vi "Actividad Extra 13 (2).vi"() -> ()   [LabVIEW 2018]
uses:
  ControlExtraTrece.ctl
panel:
  out "Toluca":bool
  out "Zinacantepec":bool
  out "Capultitlan":bool
  out "Metepec":bool
  out "San Mateo":bool
  out "KM RECORRIDOS":i32
  out "DINERO RESTANTE":i32
  out "MUNICIPIO ACTUAL":T1
  in  "Detener Recorrido":bool
  in  "Y":i32
  in  "X":i32
  # "RECORRIDO POR MUNICIPIOS"
  # "COORDENADAS"
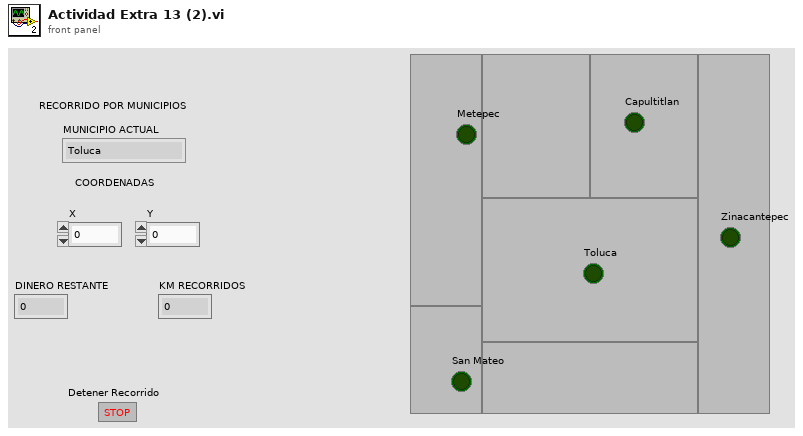
[diagram p1: front panel]
types:
  T1 = typedef "ControlExtraTrece.ctl" = enum16{"Toluca", "Metepec", "Zinacantepec", "San Mateo Atenco", "Capultitlan"}
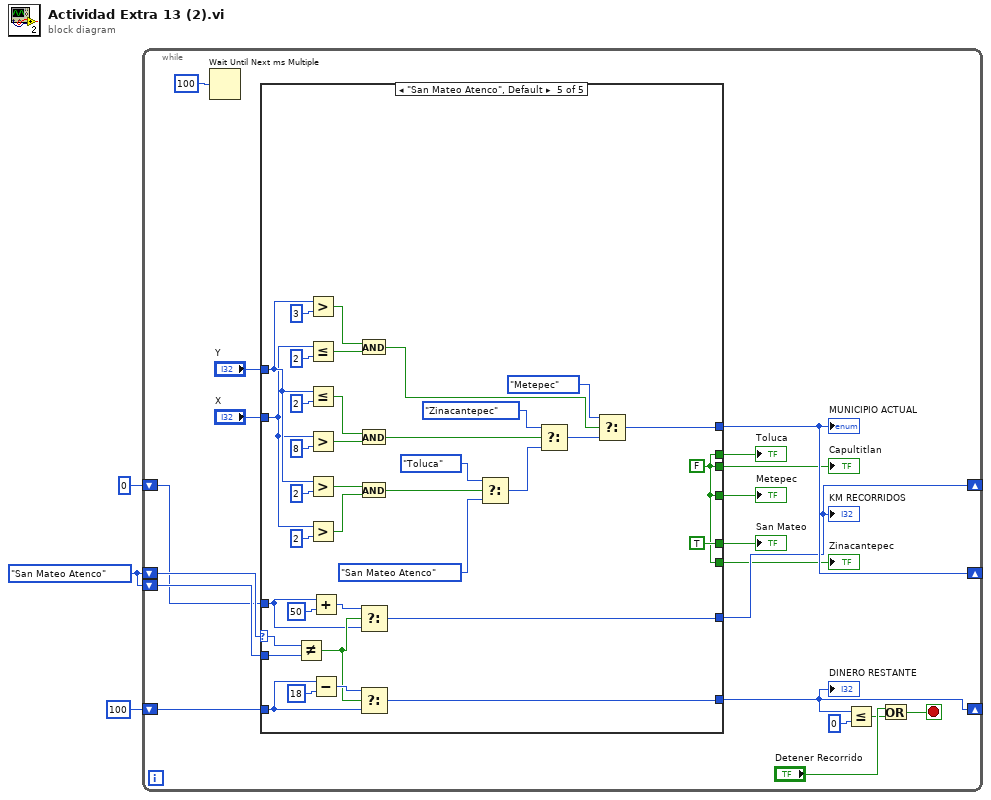
[diagram p0: block diagram]
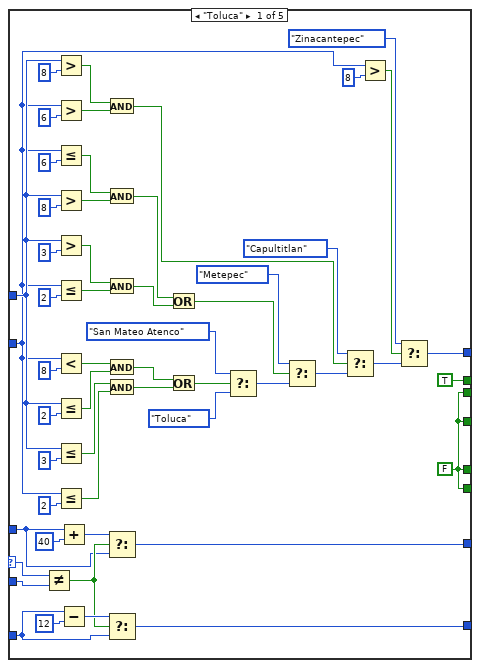
[diagram p2: hidden frame]
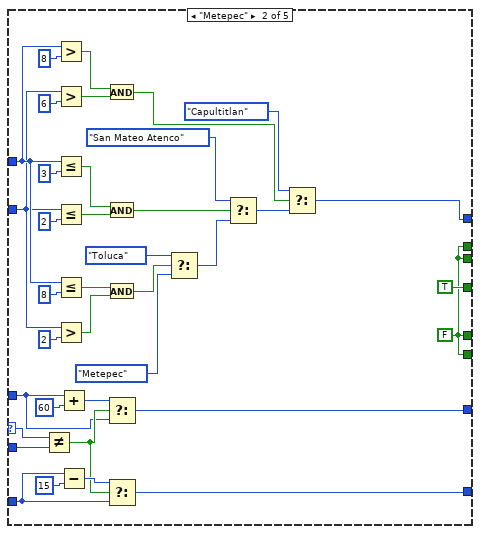
[diagram p3: hidden frame]
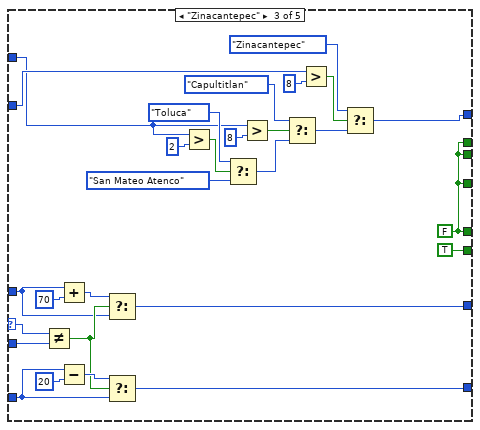
[diagram p4: hidden frame]
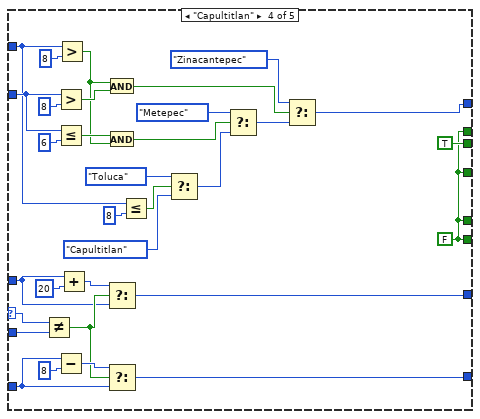
[diagram p5: hidden frame]
diagram:
  w3 = ControlExtraTrece."San Mateo Atenco"
  n1 = while {
    shift-right: [w20] -> _
    shift-left: w3 -> [w22]
    shift-left: w3 -> [w17]
    shift-right: [w10] -> _
    shift-left: 100 -> [w16]
    shift-right: [w14] -> _
    shift-left: 0 -> [w15]
    stop <- w12 stop-if-true
    n2 = Wait Until Next ms Multiple(millisecond multiple=u32 100) -> ()  [unwired: 1 out]
    n3 = case shown="\"San Mateo Atenco\", Default" w22 {
      selector: w22 -> [w25 w78 w116 w144 w175]
      tunnel: [w72 w107 w138 w167 w204] -> w20
      tunnel: "Y" -> [w45 w96 w129 w157 w193]
      tunnel: "X" -> [w43 w94 w134 w162 w190]
      tunnel: w17 -> [w36 w89 w126 w154 w186]
      tunnel: w16 -> [w34 w88 w125 w152 w182]
      tunnel: [w35 w85 w122 w153 w183] -> w10
      tunnel: w15 -> [w28 w81 w114 w147 w178]
      tunnel: [w27 w80 w118 w145 w177] -> w14
      tunnel: [w23 w76 TRUE w141 w173] -> w8
      tunnel: [w23 w76 w113 TRUE w173] -> w7
      tunnel: [w23 w76 w113 w141 TRUE] -> w6
      tunnel: [TRUE w76 w113 w141 w173] -> w5
      tunnel: [w23 TRUE w113 w141 w173] -> w4
      frame "Toluca" {
        w23 = FALSE
        n4 = Not Equal?(x=w25, y=w36) -> (x != y?=w31:bool)
        n5 = Greater?(x=w45, y=8) -> (0:w63:bool)
        n6 = Greater?(x=w43, y=6) -> (0:w62:bool)
        n7 = Less Or Equal?(x=w43, y=6) -> (x <= y?=w57:bool)
        n8 = Greater?(x=w45, y=8) -> (0:w58:bool)
        n9 = Greater?(x=w45, y=3) -> (0:w53:bool)
        n10 = Less Or Equal?(x=w43, y=2) -> (x <= y?=w54:bool)
        n11 = Less?(x=w43, y=8) -> (x < y?=w41:bool)
        n12 = Less Or Equal?(x=w45, y=2) -> (x <= y?=w40:bool)
        n13 = Less Or Equal?(x=w45, y=3) -> (x <= y?=w47:bool)
        n14 = Less Or Equal?(x=w43, y=2) -> (x <= y?=w46:bool)
        n15 = Add(x=w28, y=40) -> (x+y=w29:i32)
        n16 = Subtract(x=w34, y=12) -> (x-y=w32:i32)
        n17 = And(x=w63, y=w62) -> (x .and. y?=w61:bool)
        n18 = And(x=w57, y=w58) -> (x .and. y?=w52:bool)
        n19 = And(x=w53, y=w54) -> (x .and. y?=w51:bool)
        n20 = And(x=w41, y=w40) -> (x .and. y?=w39:bool)
        n21 = And(x=w47, y=w46) -> (x .and. y?=w38:bool)
        n22 = Select(t=w29, s=w31, f=w28) -> (s? t:f=w27:i32)
        n23 = Select(t=w32, s=w31, f=w34) -> (s? t:f=w35:i32)
        n24 = Or(x=w52, y=w51) -> (x .or. y?=w50:bool)
        n25 = Or(x=w39, y=w38) -> (x .or. y?=w37:bool)
        n26 = Select(t=ControlExtraTrece."San Mateo Atenco", s=w37, f=ControlExtraTrece."Toluca") -> (s? t:f=w75:T1)
        n27 = Select(t=ControlExtraTrece."Metepec", s=w50, f=w75) -> (s? t:f=w74:T1)
        n28 = Select(t=ControlExtraTrece."Capultitlan", s=w61, f=w74) -> (s? t:f=w73:T1)
        n29 = Greater?(x=w43, y=8) -> (0:w66:bool)
        n30 = Select(t=ControlExtraTrece."Zinacantepec", s=w66, f=w73) -> (s? t:f=w72:T1)
      }
      frame "Metepec" {
        w76 = FALSE
        n31 = Not Equal?(x=w78, y=w89) -> (x != y?=w84:bool)
        n32 = Greater?(x=w96, y=8) -> (0:w103:bool)
        n33 = Greater?(x=w94, y=6) -> (0:w104:bool)
        n34 = Less Or Equal?(x=w96, y=3) -> (x <= y?=w99:bool)
        n35 = Less Or Equal?(x=w94, y=2) -> (x <= y?=w98:bool)
        n36 = Less Or Equal?(x=w96, y=8) -> (x <= y?=w91:bool)
        n37 = Greater?(x=w94, y=2) -> (0:w92:bool)
        n38 = Add(x=w81, y=60) -> (x+y=w82:i32)
        n39 = Subtract(x=w88, y=15) -> (x-y=w86:i32)
        n40 = And(x=w103, y=w104) -> (x .and. y?=w102:bool)
        n41 = And(x=w99, y=w98) -> (x .and. y?=w97:bool)
        n42 = And(x=w91, y=w92) -> (x .and. y?=w90:bool)
        n43 = Select(t=w82, s=w84, f=w81) -> (s? t:f=w80:i32)
        n44 = Select(t=w86, s=w84, f=w88) -> (s? t:f=w85:i32)
        n45 = Select(t=ControlExtraTrece."Toluca", s=w90, f=ControlExtraTrece."Metepec") -> (s? t:f=w111:T1)
        n46 = Select(t=ControlExtraTrece."San Mateo Atenco", s=w97, f=w111) -> (s? t:f=w112:T1)
        n47 = Select(t=ControlExtraTrece."Capultitlan", s=w102, f=w112) -> (s? t:f=w107:T1)
      }
      frame "Zinacantepec" {
        w113 = FALSE
        n48 = Not Equal?(x=w116, y=w126) -> (x != y?=w121:bool)
        n49 = Add(x=w114, y=70) -> (x+y=w119:i32)
        n50 = Subtract(x=w125, y=20) -> (x-y=w123:i32)
        n51 = Select(t=w119, s=w121, f=w114) -> (s? t:f=w118:i32)
        n52 = Select(t=w123, s=w121, f=w125) -> (s? t:f=w122:i32)
        n53 = Greater?(x=w129, y=2) -> (0:w127:bool)
        n54 = Select(t=ControlExtraTrece."Toluca", s=w127, f=ControlExtraTrece."San Mateo Atenco") -> (s? t:f=w139:T1)
        n55 = Greater?(x=w129, y=8) -> (0:w130:bool)
        n56 = Select(t=ControlExtraTrece."Capultitlan", s=w130, f=w139) -> (s? t:f=w140:T1)
        n57 = Greater?(x=w134, y=8) -> (0:w132:bool)
        n58 = Select(t=ControlExtraTrece."Zinacantepec", s=w132, f=w140) -> (s? t:f=w138:T1)
      }
      frame "Capultitlan" {
        w141 = FALSE
        n59 = Not Equal?(x=w144, y=w154) -> (x != y?=w149:bool)
        n60 = Greater?(x=w162, y=8) -> (0:w164:bool)
        n61 = Less Or Equal?(x=w162, y=6) -> (x <= y?=w160:bool)
        n62 = Subtract(x=w152, y=8) -> (x-y=w150:i32)
        n63 = Greater?(x=w157, y=8) -> (0:w159:bool)
        n64 = Add(x=w147, y=20) -> (x+y=w148:i32)
        n65 = And(x=w159, y=w164) -> (x .and. y?=w163:bool)
        n66 = And(x=w160, y=w159) -> (x .and. y?=w158:bool)
        n67 = Select(t=w148, s=w149, f=w147) -> (s? t:f=w145:i32)
        n68 = Select(t=w150, s=w149, f=w152) -> (s? t:f=w153:i32)
        n69 = Less Or Equal?(x=w157, y=8) -> (x <= y?=w155:bool)
        n70 = Select(t=ControlExtraTrece."Toluca", s=w155, f=ControlExtraTrece."Capultitlan") -> (s? t:f=w171:T1)
        n71 = Select(t=ControlExtraTrece."Metepec", s=w158, f=w171) -> (s? t:f=w172:T1)
        n72 = Select(t=ControlExtraTrece."Zinacantepec", s=w163, f=w172) -> (s? t:f=w167:T1)
      }
      frame "San Mateo Atenco", Default {
        w173 = FALSE
        n73 = Not Equal?(x=w175, y=w186) -> (x != y?=w181:bool)
        n74 = Greater?(x=w193, y=3) -> (0:w200:bool)
        n75 = Less Or Equal?(x=w190, y=2) -> (x <= y?=w201:bool)
        n76 = Less Or Equal?(x=w193, y=2) -> (x <= y?=w197:bool)
        n77 = Greater?(x=w190, y=8) -> (0:w195:bool)
        n78 = Greater?(x=w193, y=2) -> (0:w189:bool)
        n79 = Greater?(x=w190, y=2) -> (0:w187:bool)
        n80 = Add(x=w178, y=50) -> (x+y=w180:i32)
        n81 = Subtract(x=w182, y=18) -> (x-y=w185:i32)
        n82 = And(x=w200, y=w201) -> (x .and. y?=w199:bool)
        n83 = And(x=w197, y=w195) -> (x .and. y?=w194:bool)
        n84 = And(x=w189, y=w187) -> (x .and. y?=w188:bool)
        n85 = Select(t=w180, s=w181, f=w178) -> (s? t:f=w177:i32)
        n86 = Select(t=w185, s=w181, f=w182) -> (s? t:f=w183:i32)
        n87 = Select(t=ControlExtraTrece."Toluca", s=w188, f=ControlExtraTrece."San Mateo Atenco") -> (s? t:f=w208:T1)
        n88 = Select(t=ControlExtraTrece."Zinacantepec", s=w194, f=w208) -> (s? t:f=w209:T1)
        n89 = Select(t=ControlExtraTrece."Metepec", s=w199, f=w209) -> (s? t:f=w204:T1)
      }
    }
    "MUNICIPIO ACTUAL" <- w20
    "DINERO RESTANTE" <- w10
    "KM RECORRIDOS" <- w14
    "Zinacantepec" <- w8
    "Capultitlan" <- w7
    "San Mateo" <- w6
    "Toluca" <- w5
    "Metepec" <- w4
    n90 = Less Or Equal?(x=w10, y=0) -> (x <= y?=w11:bool)
    n91 = Or(x="Detener Recorrido", y=w11) -> (x .or. y?=w12:bool)
  }
